vi "Get External Sensor Data.vi"(8 "error in (no error)":errorcluster) -> (0 "error out":errorcluster, 1 "Offsets":dbl[](array[numeric]), 2 "Data Out":dbl[](array[numeric]), 3 "Volts":dbl[](array[numeric]))   [LabVIEW 2009]
uses:
  Data Access Objects/Metadata/DAO Actions.ctl
  Data Access Objects/Metadata/DAO Actions with Remove.ctl
  Transactions/Dataset Transaction Id.ctl
  Transactions/Dataset Source.ctl
  Transactions/Dataset Type.ctl
  Apps/Yes No Button.ctl
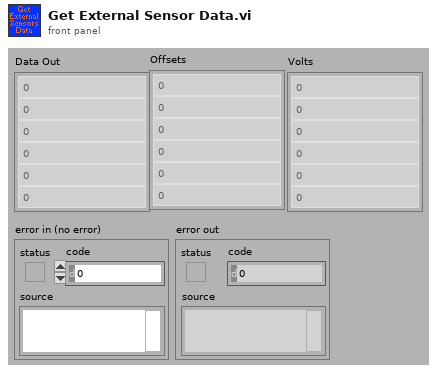
[diagram p1: front panel]
types:
  T1 = typedef "Yes No Button.ctl" = bool
  T2 = typedef "Dataset Transaction Id.ctl" = cluster{"Dataset Source":T3, "Dataset Type":T4, "Hold":T1, "Volts":T1, "Tag":string}
  T3 = typedef "Dataset Source.ctl" = enum16{"LBCB 1", "LBCB 2", "Combined", "External Sensors"}
  T4 = typedef "Dataset Type.ctl" = enum16{"LVDT", "Load Cell", "Actuator Command", "Servo Error", "Displacement Command", "Displacement", "Force"}
  T5 = typedef "DAO Actions with Remove.ctl" = enum16{"Init", "Get", "Set", "Remove"}
  T6 = typedef "DAO Actions.ctl" = enum16{"Init", "Get", "Set"}
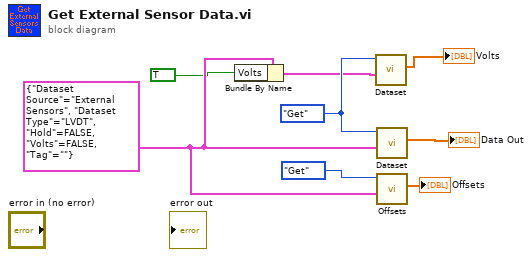
[diagram p0: block diagram]
diagram:
  w3 = T2 {"Dataset Source"=enum."External Sensors", "Dataset Type"=enum."LVDT", "Hold"=FALSE, "Volts"=FALSE, "Tag"=""} ("Dataset Trans Id")
  w5 = DAO_Actions."Get" ("DAO Actions")
  n1 = Bundle By Name(cluster=w3, "Volts"=T1 TRUE) -> (w1:T2)
  n2 = call "Dataset.vi"("Dataset Trans Id"=w1, "DAO Actions"=w5) -> ("Data Out"=→"Volts":dbl[])  [unwired: 8 in, 1 out]
  n3 = call "Dataset.vi"("Dataset Trans Id"=w3, "DAO Actions"=w5) -> ("Data Out"=→"Data Out":dbl[])  [unwired: 8 in, 1 out]
  n4 = call "Offsets.vi"("Dataset Trans Id"=w3, "DAO Actions"=DAO_Actions_with_Remove."Get") -> ("Data Out"=→"Offsets":dbl[])  [unwired: 7 in, 2 out]
